vi "StateHistory.vi"(11 "Current State in":string) -> (2 "Current State out":string, 3 "delimited string":string)   [LabVIEW 2016]
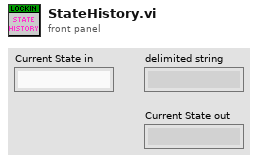
[diagram p1: front panel]
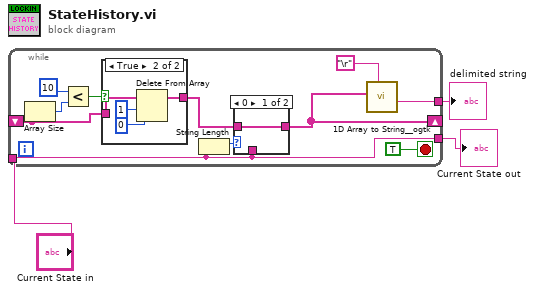
[diagram p0: block diagram]
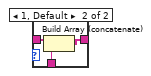
[diagram p2: hidden frame]
diagram:
  n1 = while {
    tunnel: [w14] -> w1
    tunnel: "Current State in" -> [w6]
    tunnel: [w6] -> w3
    shift-right: [w5] -> _
    shift-left: _ -> [w4]
    stop <- TRUE stop-if-true
    n2 = Array Size(array=w4) -> (size(s)=w11:i32)
    n3 = Less?(x=10 ("length"), y=w11) -> (x < y?=w13:bool)
    n4 = case shown="True" w13 {
      tunnel: w4 -> [w19 w20]
      tunnel: [w19 w22] -> w12
      frame False {
      }
      frame True {
        n5 = Delete From Array(array=w20, length=1, index=0) -> (array with subset deleted=w22:string[])  [unwired: 1 out]
      }
    }
    n6 = String Length(string=w6) -> (length=w10:i32)
    n7 = case shown="0" w10 {
      tunnel: w12 -> [w15 w18]
      tunnel: [w15 w17] -> w5
      tunnel: w6 -> [_ w16]
      frame 0 {
      }
      frame 1, Default {
        n8 = Build Array (concatenate)(w18, w16) -> (w17:string[])
      }
    }
    n9 = call <userlib>:"1D Array to String__ogtk.vi"("delimiter (Tab)"="\r", "Array of Strings"=w5) -> ("delimited string"=w14:string)  [unwired: 9 in]
  }
  "Current State out" <- w3
  "delimited string" <- w1
